vi "test-AttrMap-ImportValue.vi"(8 "error in (no error)":errorcluster, 11 "TestCase in":refnum<class "MyTestCase.lvclass">) -> (0 "error out":errorcluster, 3 "TestCase out":refnum<class "MyTestCase.lvclass">)   [LabVIEW 2019, in "MyTestCase.lvclass"]
uses:
  MyTestCase.lvclass
  <vilib>/addons/_JKI Toolkits/VI Tester/TestCase.llb/TestCase.lvclass
  lv-apt-json-file.lvlib
  C:/Program Files (x86)/National Instruments/LabVIEW 2019/vi.lib/addons/_JKI Toolkits/VI Tester/TestCase.llb/TestCase.lvclass
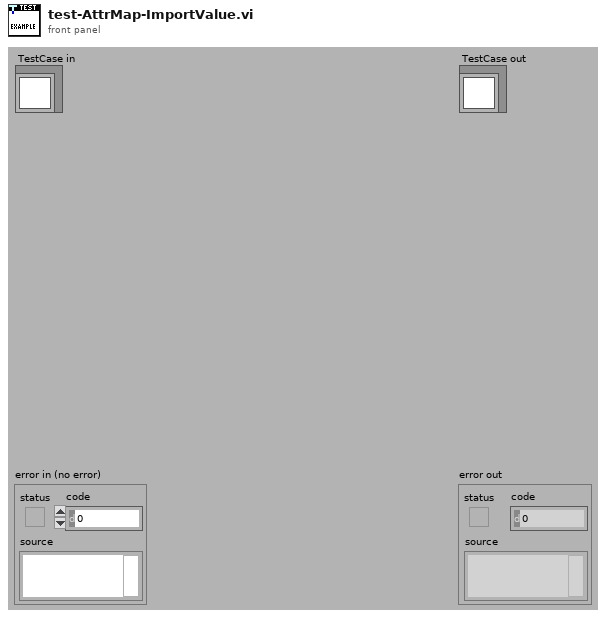
[diagram p1: front panel]
types:
  T1 = cluster{"nUmeric":i32, "string":string, "Cluster":cluster{"numeric":i32, "string":string, "cluster":cluster{"numeric":i32, "string":string, "cluster":cluster{"numeric":i32, "string":string}}}}
  T2 = typedef "lv-apt-json-file.lvlib/Def-AttrMap.ctl" = cluster{"Map":variant}
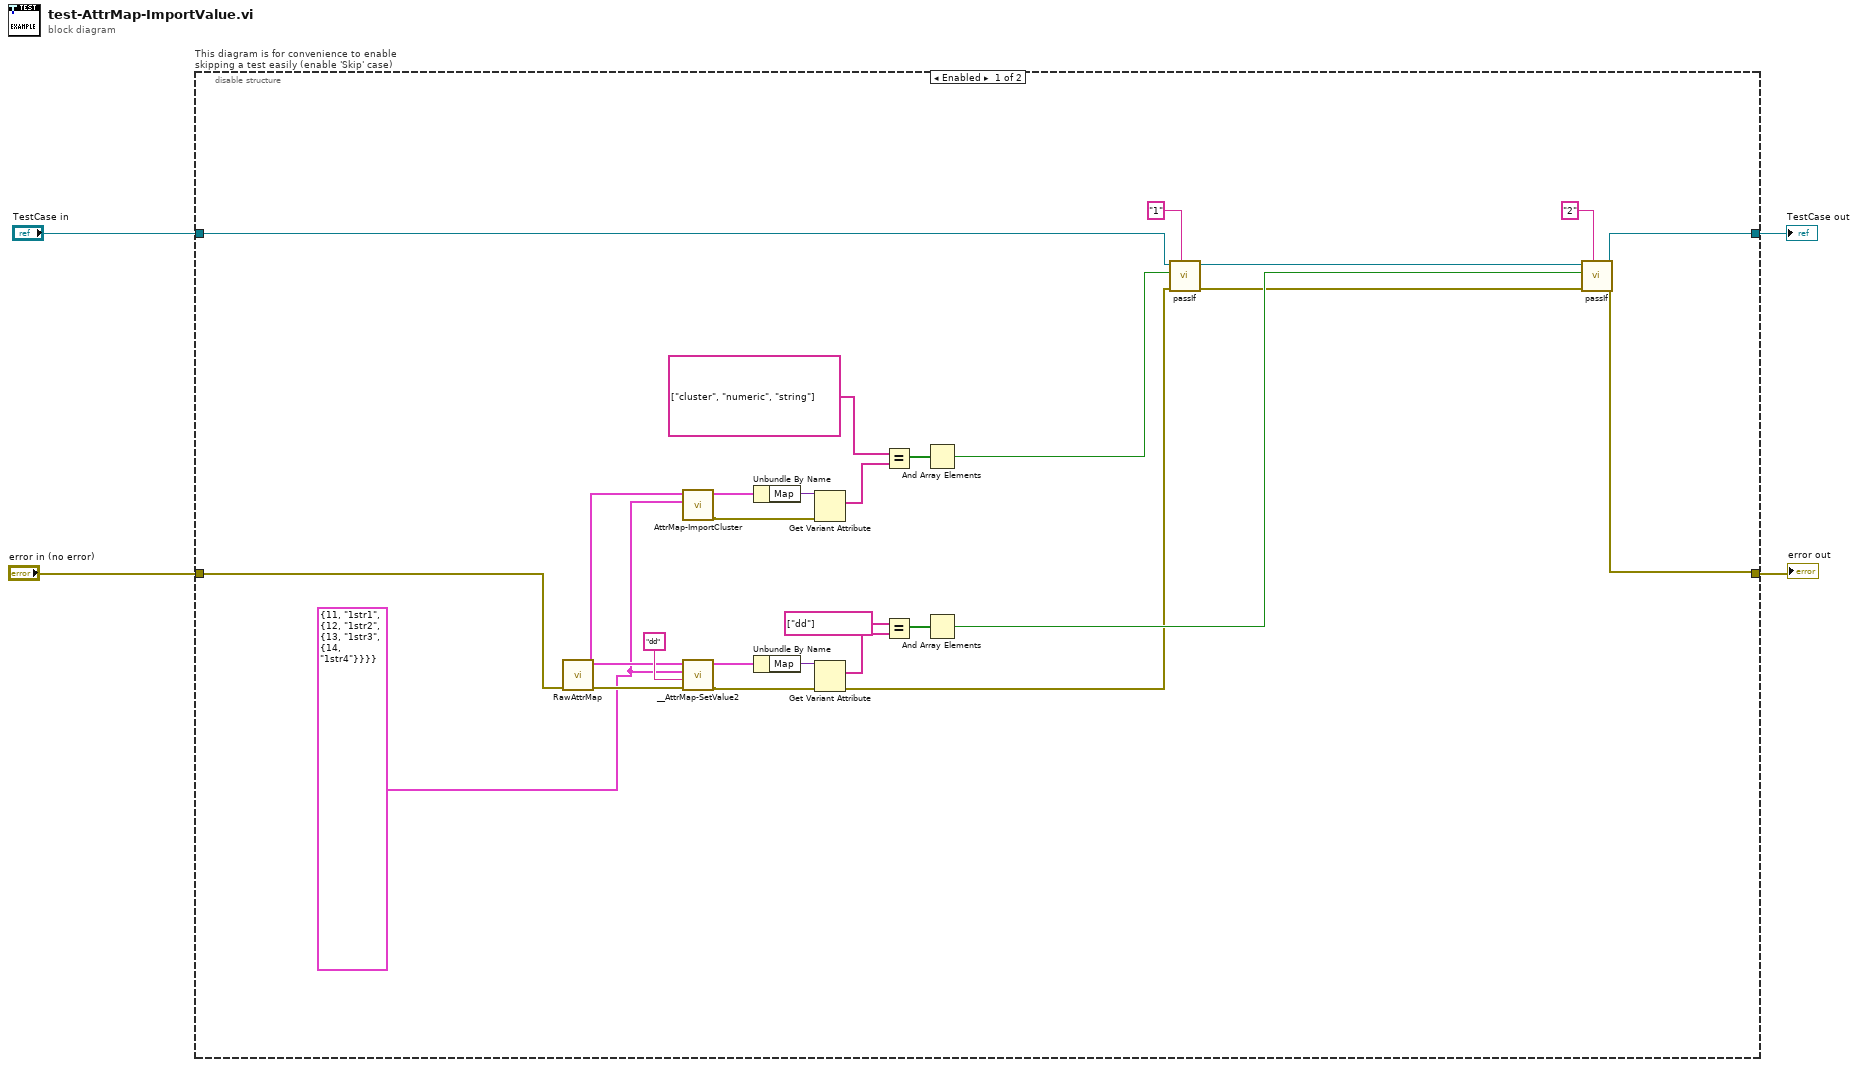
[diagram p0: block diagram]
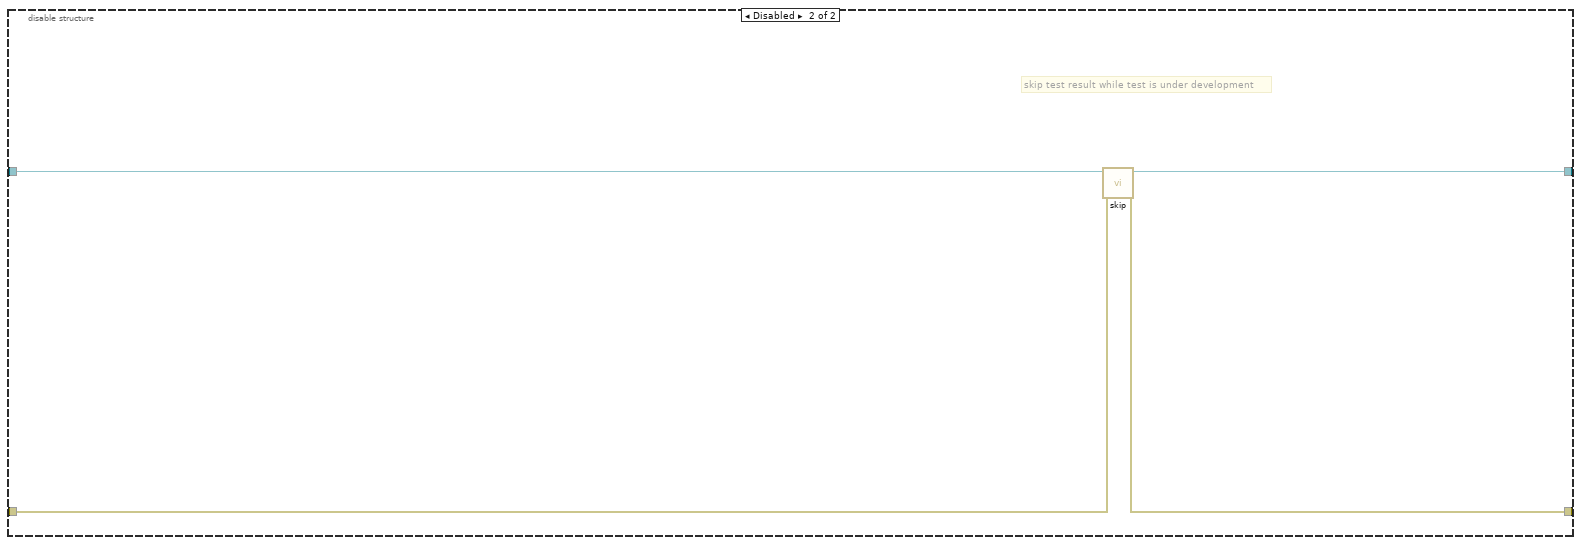
[diagram p2: hidden frame]
diagram:
  n1 = disable-structure "This diagram is for convenience to enable skipping a test easily (enable 'Skip' case)" shown="Enabled" {
    disable-tunnel: "TestCase in" -> [w10 w34]
    disable-tunnel: [w30 w32] -> w1
    disable-tunnel: [w29 w33] -> w3
    disable-tunnel: "error in (no error)" -> [w27 w31]
    frame Enabled {
      w12 = T1 {"nUmeric"=11, "string"="1str1", "Cluster"={"numeric"=12, "string"="1str2", "cluster"={"numeric"=13, "string"="1str3", "cluster"={"numeric"=14, "string"="1str4"}}}} ("Cluster")
      n2 = call "RawAttrMap.vi"() -> ("AttrMap"=w13:T2)  [unwired: 11 in]
      n3 = call "AttrMap-ImportCluster.vi"("Cluster"=w12, "AttrMap in"=w13) -> ("error out"=w14:errorcluster, "AttrMap out"=w15:T2)  [unwired: 8 in]
      n4 = call "__AttrMap-SetValue2.vi"("error in (no error)"=w27, "Key"="dd", "Value"=w12, "AttrMap in"=w13) -> ("error out"=w26:errorcluster, "AttrMap out"=w25:T2)  [unwired: 6 in]
      n5 = Unbundle By Name(w15) -> ("Map"=w16:variant)
      n6 = Unbundle By Name(w25) -> ("Map"=w24:variant)
      n7 = Get Variant Attribute(Variant=w16, error in=w14) -> (names=w17:string[])  [unwired: 2 in, 3 out]
      n8 = Get Variant Attribute(Variant=w24, error in=w26) -> (names=w23:string[], error out=w7:errorcluster)  [unwired: 2 in, 2 out]
      n9 = Equal?(x=string[] ["cluster", "numeric", "string"], y=w17) -> (x = y?=w19:bool[])
      n10 = Equal?(x=string[] ["dd"], y=w23) -> (x = y?=w21:bool[])
      n11 = And Array Elements(Boolean array=w19) -> (logical AND=w11:bool)
      n12 = And Array Elements(Boolean array=w21) -> (logical AND=w20:bool)
      n13 = call-dynamic "passIf.vi"("custom report message (\"\")"="1" ("custom report message (\"\")"), "error in (no error)"=w7, "pass"=w11, "TestCase in"=w10) -> ("error out"=w8:errorcluster, "TestCase out"=w9:refnum<class "MyTestCase.lvclass">)  [unwired: 6 in]
      n14 = call-dynamic "passIf.vi"("custom report message (\"\")"="2" ("custom report message (\"\")"), "error in (no error)"=w8, "pass"=w20, "TestCase in"=w9) -> ("error out"=w29:errorcluster, "TestCase out"=w30:refnum<class "MyTestCase.lvclass">)  [unwired: 6 in]
    }
    frame Disabled {
      # "skip test result while test is under development"
      n15 = call <vilib>:"skip.vi"("error in (no error)"=w31, "TestCase in"=w34) -> ("error out"=w33:errorcluster, "TestCase out"=w32:refnum<class "MyTestCase.lvclass">)  [unwired: 8 in]
    }
  }
  "error out" <- w3
  "TestCase out" <- w1
